vi "TicVariableReference.vi"(9 "Variable":string(combo)) -> (1 "VariableDescription":T1 {"Offset" format="%02x"}, 3 "VariablesDescriptor":T1[](array[typedef]) {"Offset" format="%02x"})   [LabVIEW 2018]
uses:
  VariableDescriptor.ctl
  <vilib>/Utility/file.llb/Read Delimited Spreadsheet (string).vi
panel:
  out "file path":path
  out "all rows":string[][](table)
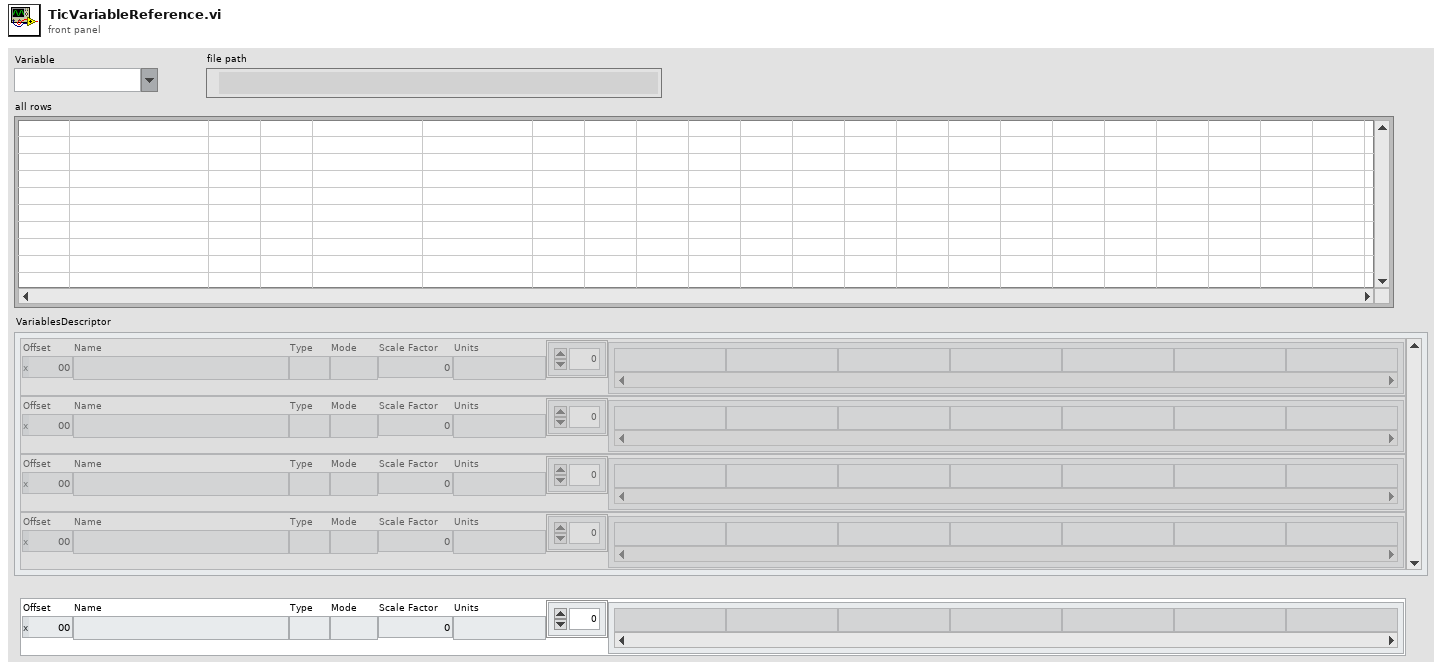
[diagram p1: front panel]
types:
  T1 = typedef "VariableDescriptor.ctl" = cluster{"Offset":u8, "Name":string, "Type":string, "Mode":string, "Scale Factor":dbl, "Units":string, "Coding":string[]}
  T2 = cluster{"Offset":u8, "Name":string, "Type":string, "Mode":string, "Scale Factor":dbl, "Units":string, "Coding":string[]}
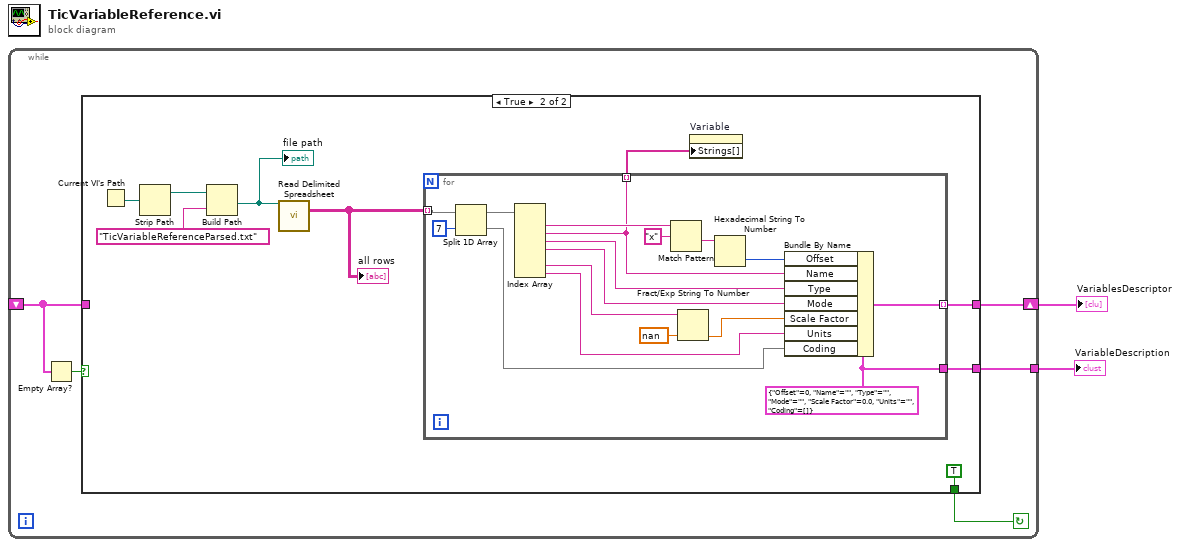
[diagram p0: block diagram]
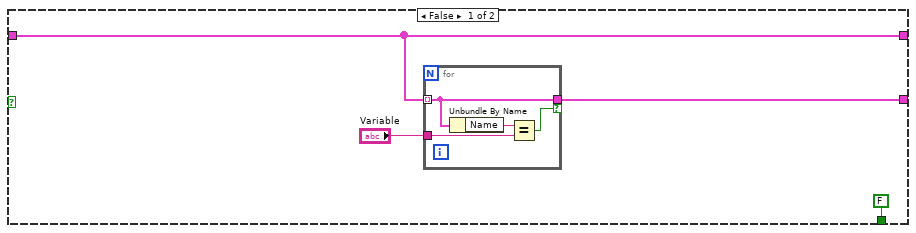
[diagram p2: hidden frame]
diagram:
  n1 = while {
    shift-right: [w7] -> w2
    shift-left: _ -> [w4]
    tunnel: [w3] -> w1
    stop <- w5 continue-if-true
    n2 = Empty Array?(array=w4) -> (empty?=w6:bool)
    n3 = case shown="True" w6 {
      tunnel: [w9 w18] -> w7
      tunnel: [FALSE TRUE] -> w5
      tunnel: w4 -> [w9 _]
      tunnel: [w8 w16] -> w3
      frame False {
        n4 = for {
          tunnel: w9 -> [w13] mode=indexing
          tunnel: "Variable" -> [w15]
          tunnel: [w13] -> w8 if=w12
          n5 = Unbundle By Name(w13) -> ("Name"=w14:string)
          n6 = Equal?(x=w14, y=w15) -> (x = y?=w12:bool)
        }
      }
      frame True {
        n7 = Current VI's Path() -> (path=w22:path)
        n8 = Strip Path(path=w22) -> (stripped path=w21:path)  [unwired: 1 out]
        n9 = Build Path(base path=w21, name or relative path="TicVariableReferenceParsed.txt") -> (appended path=w19:path)
        "file path" <- w19
        n10 = call-poly <vilib>:"Read Delimited Spreadsheet.vi"("file path (dialog if empty)"=w19) -> ("all rows"=w24:string[][])  [unwired: 9 in, 5 out]
        "all rows" <- w24
        n11 = for {
          tunnel: w24 -> [w31] mode=indexing
          tunnel: [w26] -> w18 mode=indexing
          tunnel: [w27] -> w23 mode=indexing
          tunnel: [w25] -> w16
          w25 = T2 {"Offset"=0, "Name"="", "Type"="", "Mode"="", "Scale Factor"=0.0, "Units"="", "Coding"=[]} ("Cluster")
          n12 = Split 1D Array(array=w31, index=7) -> (first subarray=w30:string[], second subarray=w28:string[])
          n13 = Index Array(array=w30) -> (element #1=w40:string, element #2=w27:string, element #3=w37:string, element #4=w36:string, element #6=w33:string, element #7=w32:string)  [unwired: 7 in, 1 out]
          n14 = Match Pattern(string=w40, regular expression="x") -> (after substring=w39:string)  [unwired: 1 in, 3 out]
          n15 = Fract/Exp String To Number(string=w33, default (0 dbl)=nan ("default (0 DBL)")) -> (number=w35:dbl)  [unwired: 2 in, 1 out]
          n16 = Hexadecimal String To Number(string=w39) -> (number=w41:u32)  [unwired: 2 in, 1 out]
          n17 = Bundle By Name(cluster=w25, "Offset"=w41, "Name"=w27, "Type"=w37, "Mode"=w36, "Scale Factor"=w35, "Units"=w32, "Coding"=w28) -> (w26:T2)
        }
        n18 = property on="Variable" class="CmbBox"("Strings[]"=w23) -> ()  [unwired: 2 in, 2 out]
      }
    }
  }
  "VariableDescription" <- w1
  "VariablesDescriptor" <- w2
